vi "GetDictionary.vi"(8 "error in (no error)":errorcluster caption="Fehler (Eingang, kein Fehler)", 11 "PassDataAround Eingang":refnum<class "PassDataAround.lvclass"> caption="DNL_LabVIEW Object in") -> (0 "error out":errorcluster caption="Fehler (Ausgang)", 2 "LvDictionary.lvlib:DictionaryString.lvclass":refnum<class "DictionaryString.lvclass">, 3 "PassDataAround Ausgang":refnum<class "PassDataAround.lvclass"> caption="DNL_LabVIEW Object out")   [LabVIEW 2013, in "PassDataAround.lvlib" / "PassDataAround.lvclass"]
uses:
  PassDataAround.lvclass
  LvDictionary/DictionaryStringClass/DictionaryString.lvclass
  PassDataAround.lvclass/PassDataAround.ctl
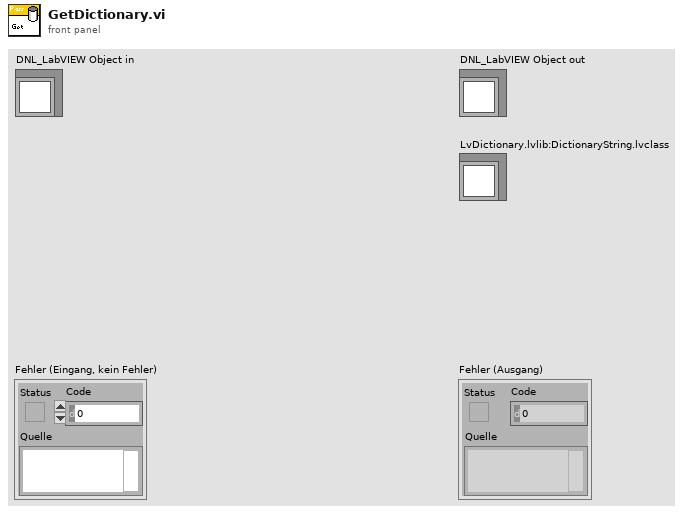
[diagram p1: front panel]
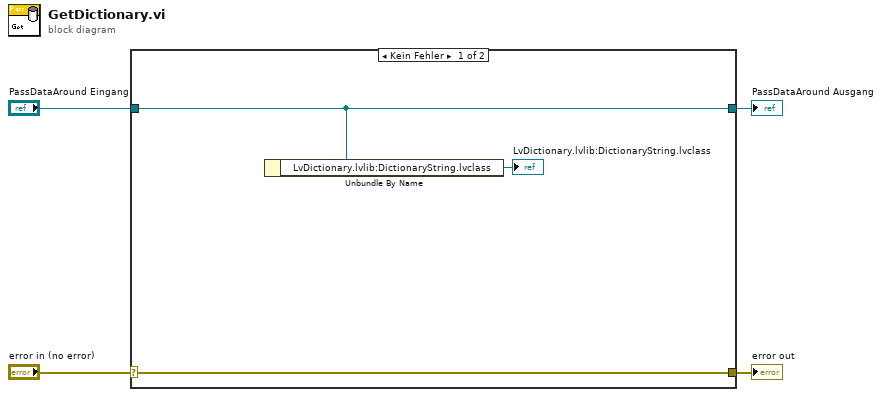
[diagram p0: block diagram]
diagram:
  n1 = case shown="Kein Fehler" "error in (no error)" {
    selector: "error in (no error)" -> [w7 w9]
    tunnel: [w7 w9] -> w3
    tunnel: [w6 w8] -> w1
    tunnel: "PassDataAround Eingang" -> [w6 w8]
    frame No Error {
      n2 = Unbundle By Name(w6) -> ("LvDictionary.lvlib:DictionaryString.lvclass"=→"LvDictionary.lvlib:DictionaryString.lvclass":refnum<class "DictionaryString.lvclass">)
    }
    frame Error {
    }
  }
  "error out" <- w3
  "PassDataAround Ausgang" <- w1
